vi "Build Path.vi"(8 "error in (no error)":errorcluster, 10 "Path":string, 11 "IPath Builder in":refnum<class "IPath Builder.lvclass">) -> (0 "error out":errorcluster, 3 "Path":path)   [LabVIEW 2020, in "Test Executive.lvlib" / "IPath Builder.lvclass"]
uses:
  <vilib>/gpm_packages/@cs/test-executive/Source/Path Builder/IPath Builder/IPath Builder.lvclass
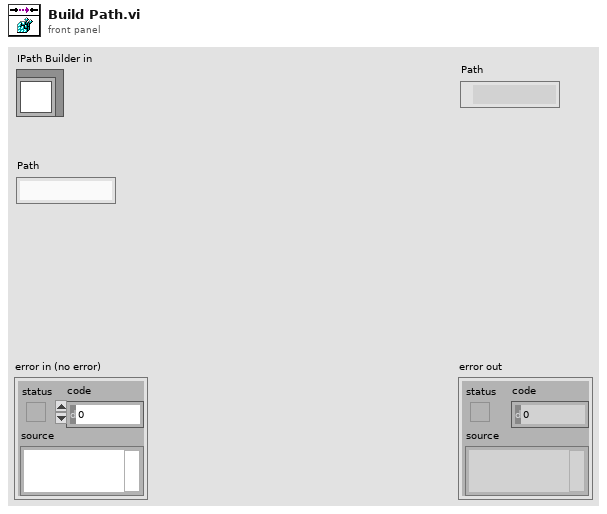
[diagram p1: front panel]
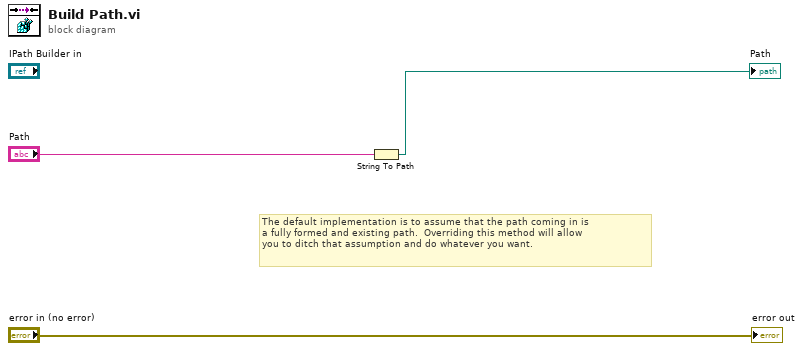
[diagram p0: block diagram]
diagram:
  # "The default implementation is to assume that the path coming in is\na fully formed and existing path.  Overriding this method will allow\nyou to ditch that assumption and do whatever you want."
  n1 = String To Path(string="Path") -> (path=→"Path":path)
  "error out" <- "error in (no error)"
